vi "circuits-resistor.vi"(1 "Invert Y":bool, 2 "Invert X":bool, 5 "L2":dbl=0.1, 6 "Swap-XY":bool, 7 "L1":dbl=0.1, 8 "Device in Y":refnum<k24>, 9 "GetPOS Y":refnum<vi>, 10 "GetPOS X":refnum<vi>, 11 "Device in X":refnum<k24>) -> (0 "Device out Y":refnum<k24>, 3 "Device out X":refnum<k24>)   [LabVIEW 2014]
doc: "André Romero - 2019\nandretec@ifsc.usp.br"
uses:
  C:/user-Lab/AndreTec/GITs/andretec/Thorlabs-Vector-Move/kinesisTec/Kinesis/Thorlabs.MotionControl.TCube.DCServoCLI.dll
  kinesisTec/Kinesis/Thorlabs.MotionControl.TCube.DCServoCLI.dll
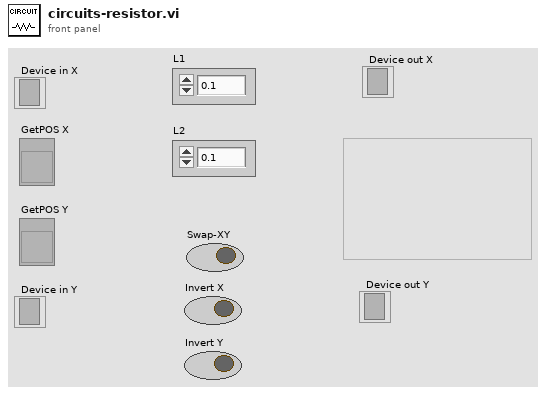
[diagram p1: front panel]
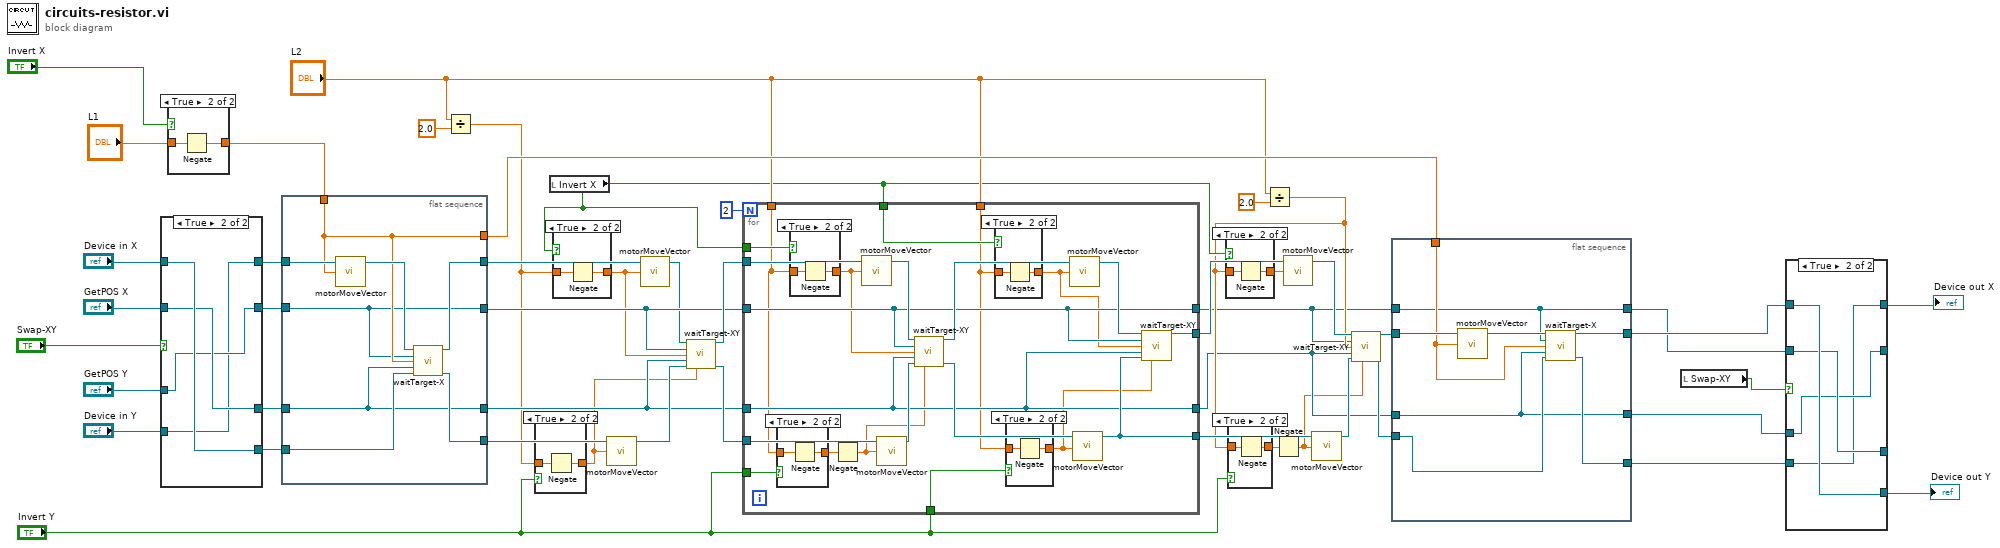
[diagram p0: block diagram]
diagram:
  n1 = case shown="True" "Swap-XY" {
    tunnel: "Device in X" -> [w51 w57]
    tunnel: [w51 w54] -> w30
    tunnel: "GetPOS Y" -> [w53 w55]
    tunnel: [w53 w56] -> w28
    tunnel: "Device in Y" -> [w52 w54]
    tunnel: [w52 w57] -> w26
    tunnel: "GetPOS X" -> [w50 w56]
    tunnel: [w50 w55] -> w24
    frame False {
    }
    frame True {
    }
  }
  n2 = case shown="True" "Invert X" {
    tunnel: "L1" -> [w58 w60]
    tunnel: [w58 w59] -> w21
    frame False {
    }
    frame True {
      n3 = Negate(x=w60) -> (-x=w59:dbl)
    }
  }
  n4 = flat-sequence {
    tunnel: w30 -> [w68]
    tunnel: [w65] -> w33
    tunnel: w26 -> [w66]
    tunnel: [w64] -> w46
    tunnel: [w62] -> w42
    tunnel: [w61] -> w41
    tunnel: [w63] -> w49
    tunnel: w21 -> [w63]
    tunnel: w24 -> [w62]
    tunnel: w28 -> [w61]
    frame #0 {
      n5 = call "motorMoveVector.vi"("Distance"=w63, "Device in"=w68) -> ("Device out"=w67:refnum<k24>)  [unwired: 3 in]
      n6 = call "waitTarget-X.vi"("Device in X"=w67, "GetPOS X"=w62, "Position X"=w63, "GetPOS Y"=w61, "Device in Y"=w66) -> ("Device out X"=w65:refnum<k24>, "Device out Y"=w64:refnum<k24>)  [unwired: 7 in, 2 out]
    }
  }
  n7 = Divide(x="L2", y=2.0) -> (x/y=w15:dbl)
  n8 = case shown="True" "Invert Y" {
    tunnel: w15 -> [w69 w71]
    tunnel: [w69 w70] -> w9
    frame False {
    }
    frame True {
      n9 = Negate(x=w71) -> (-x=w70:dbl)
    }
  }
  n10 = local read "Invert X"() -> (w16:bool)
  n11 = case shown="True" w16 {
    tunnel: [w72 w73] -> w19
    tunnel: w15 -> [w72 w74]
    frame False {
    }
    frame True {
      n12 = Negate(x=w74) -> (-x=w73:dbl)
    }
  }
  n13 = call "motorMoveVector.vi"("Distance"=w9, "Device in"=w46) -> ("Device out"=w45:refnum<k24>)  [unwired: 3 in]
  n14 = call "motorMoveVector.vi"("Distance"=w19, "Device in"=w33) -> ("Device out"=w32:refnum<k24>)  [unwired: 3 in]
  n15 = call "waitTarget-XY.vi"("Device in X"=w32, "GetPOS X"=w42, "Position X"=w19, "GetPOS Y"=w41, "Device in Y"=w45, "Position Y"=w9) -> ("Device out X"=w47:refnum<k24>, "Device out Y"=w44:refnum<k24>)  [unwired: 6 in, 2 out]
  n16 = for {
    N: 2 -> [_]
    tunnel: w47 -> [w95]
    tunnel: w44 -> [w94]
    tunnel: [w89] -> w40
    tunnel: [w88] -> w39
    tunnel: w42 -> [w87]
    tunnel: w41 -> [w86]
    tunnel: "L2" -> [w80]
    tunnel: [w87] -> w11
    tunnel: [w86] -> w10
    tunnel: "L2" -> [w78]
    tunnel: w16 -> [w85]
    tunnel: w16 -> [w82]
    tunnel: "Invert Y" -> [w79]
    tunnel: "Invert Y" -> [w77]
    n17 = case shown="True" w79 {
      tunnel: [w100 w101] -> w81
      tunnel: w80 -> [w100 w102]
      frame False {
      }
      frame True {
        n18 = Negate(x=w102) -> (-x=w101:dbl)
      }
    }
    n19 = case shown="True" w85 {
      tunnel: w80 -> [w106 w108]
      tunnel: [w106 w107] -> w84
      frame False {
      }
      frame True {
        n20 = Negate(x=w108) -> (-x=w107:dbl)
      }
    }
    n21 = Negate(x=w81) -> (-x=w76:dbl)
    n22 = call "motorMoveVector.vi"("Distance"=w84, "Device in"=w95) -> ("Device out"=w93:refnum<k24>)  [unwired: 3 in]
    n23 = call "motorMoveVector.vi"("Distance"=w76, "Device in"=w94) -> ("Device out"=w96:refnum<k24>)  [unwired: 3 in]
    n24 = call "waitTarget-XY.vi"("Device in X"=w93, "GetPOS X"=w87, "Position X"=w84, "GetPOS Y"=w86, "Device in Y"=w96, "Position Y"=w76) -> ("Device out X"=w92:refnum<k24>, "Device out Y"=w91:refnum<k24>)  [unwired: 6 in, 2 out]
    n25 = case shown="True" w82 {
      tunnel: [w103 w104] -> w83
      tunnel: w78 -> [w103 w105]
      frame False {
      }
      frame True {
        n26 = Negate(x=w105) -> (-x=w104:dbl)
      }
    }
    n27 = case shown="True" w77 {
      tunnel: [w97 w98] -> w75
      tunnel: w78 -> [w97 w99]
      frame False {
      }
      frame True {
        n28 = Negate(x=w99) -> (-x=w98:dbl)
      }
    }
    n29 = call "motorMoveVector.vi"("Distance"=w83, "Device in"=w92) -> ("Device out"=w90:refnum<k24>)  [unwired: 3 in]
    n30 = call "motorMoveVector.vi"("Distance"=w75, "Device in"=w91) -> ("Device out"=w88:refnum<k24>)  [unwired: 3 in]
    n31 = call "waitTarget-XY.vi"("Device in X"=w90, "GetPOS X"=w87, "Position X"=w83, "GetPOS Y"=w86, "Device in Y"=w88, "Position Y"=w75) -> ("Device out X"=w89:refnum<k24>)  [unwired: 6 in, 3 out]
  }
  n32 = Divide(x="L2", y=2.0) -> (x/y=w14:dbl)
  n33 = case shown="True" w16 {
    tunnel: [w109 w110] -> w17
    tunnel: w14 -> [w109 w111]
    frame False {
    }
    frame True {
      n34 = Negate(x=w111) -> (-x=w110:dbl)
    }
  }
  n35 = case shown="True" "Invert Y" {
    tunnel: w14 -> [w112 w114]
    tunnel: [w112 w113] -> w13
    frame False {
    }
    frame True {
      n36 = Negate(x=w114) -> (-x=w113:dbl)
    }
  }
  n37 = Negate(x=w13) -> (-x=w8:dbl)
  n38 = call "motorMoveVector.vi"("Distance"=w17, "Device in"=w40) -> ("Device out"=w38:refnum<k24>)  [unwired: 3 in]
  n39 = call "motorMoveVector.vi"("Distance"=w8, "Device in"=w39) -> ("Device out"=w37:refnum<k24>)  [unwired: 3 in]
  n40 = call "waitTarget-XY.vi"("Device in X"=w38, "GetPOS X"=w11, "Position X"=w14, "GetPOS Y"=w10, "Device in Y"=w37, "Position Y"=w8) -> ("Device out X"=w35:refnum<k24>, "Device out Y"=w34:refnum<k24>)  [unwired: 6 in, 2 out]
  n41 = flat-sequence {
    tunnel: w35 -> [w122]
    tunnel: w34 -> [w118]
    tunnel: [w117] -> w5
    tunnel: w10 -> [w115]
    tunnel: w49 -> [w120]
    tunnel: [w119] -> w6
    tunnel: w11 -> [w116]
    tunnel: [w116] -> w4
    tunnel: [w115] -> w3
    frame #0 {
      n42 = call "motorMoveVector.vi"("Distance"=w120, "Device in"=w122) -> ("Device out"=w121:refnum<k24>)  [unwired: 3 in]
      n43 = call "waitTarget-X.vi"("Device in X"=w121, "GetPOS X"=w116, "Position X"=w120, "GetPOS Y"=w115, "Device in Y"=w118) -> ("Device out X"=w119:refnum<k24>, "Device out Y"=w117:refnum<k24>)  [unwired: 7 in, 2 out]
    }
  }
  n44 = local read "Swap-XY"() -> (w7:bool)
  n45 = case shown="True" w7 {
    tunnel: w6 -> [w124 w130]
    tunnel: [w124 w127] -> w1
    tunnel: w3 -> [w126 w128]
    tunnel: [w126 w129] -> _
    tunnel: w5 -> [w125 w127]
    tunnel: [w125 w130] -> w2
    tunnel: w4 -> [w123 w129]
    tunnel: [w123 w128] -> _
    frame False {
    }
    frame True {
    }
  }
  "Device out X" <- w1
  "Device out Y" <- w2
